vi "Log Errors.vi"(8 "error in (no error)":errorcluster, 11 "SV B-M (Host) in":refnum<class "SV B-M (Host).lvclass">) -> (0 "error out":errorcluster)   [LabVIEW 2015, in "SV B-M (Host).lvclass"]
doc: "Create an error log text file in the test directory that follows a template to record any error that occured during the benchmark sequence. If the error is known or expected, describe the error in detail."
uses:
  SV B-M (Host).lvclass
  SV B-M (Host).lvclass/SV B-M (Host).ctl
  Listbox - In Progress.vi
  Listbox - Complete.vi
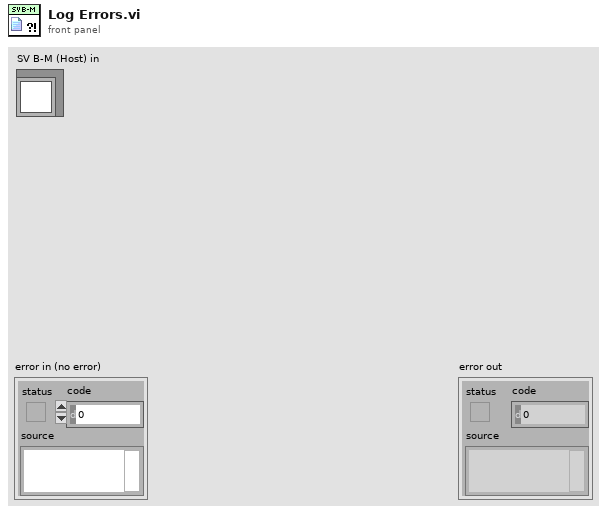
[diagram p1: front panel]
types:
  T1 = enum16{"open", "replace", "create", "open or create", "replace or create", "replace or create with confirmation"}
  T2 = typedef "Target Type.ctl" = enum16{"cRIO-9012", "cRIO-9014", "cRIO-9022", "cRIO-9023", "cRIO-9024", "cRIO-9025", "cRIO-9068", "cRIO-9073", "cRIO-9074", "cRIO-9075", "cRIO-9076", "cRIO-9081", "cRIO-9082", "myRIO-1900", "myRIO-1950", "PXI-8101", "PXI-8115", "PXI-8119", "PXI-8820", "PXIe-8100", "PXIe-8101", "PXIe-8133", "PXIe-8135", "PXIe-8820", "sbRIO-9605", "sbRIO-9606", "sbRIO-9623", "sbRIO-9626", "sbRIO-9633", "sbRIO-9636", "Unlisted (Linux-RT)", "Unlisted (PharLap)", "Unlisted (VxWorks)", "Windows Target"}
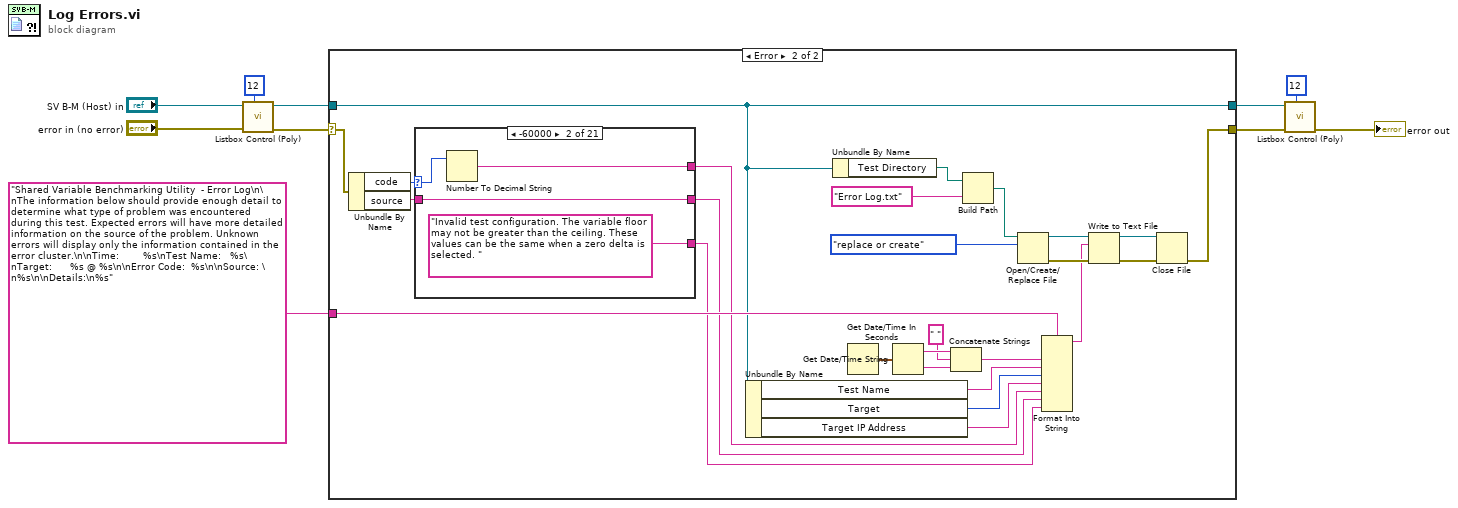
[diagram p0: block diagram]
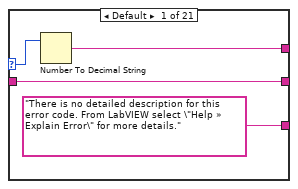
[diagram p3: hidden frame]
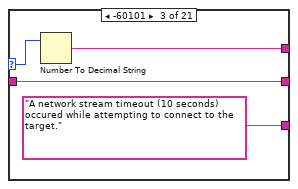
[diagram p4: hidden frame]
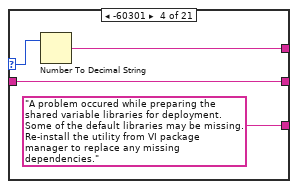
[diagram p5: hidden frame]
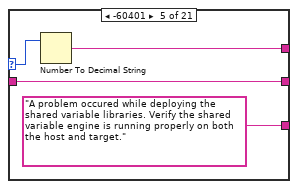
[diagram p6: hidden frame]
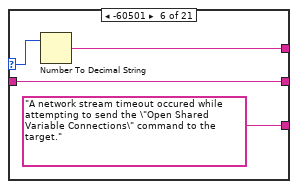
[diagram p7: hidden frame]
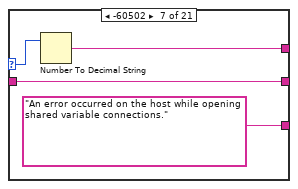
[diagram p8: hidden frame]
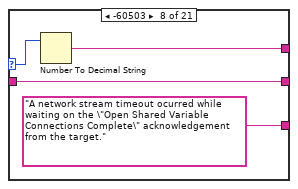
[diagram p9: hidden frame]
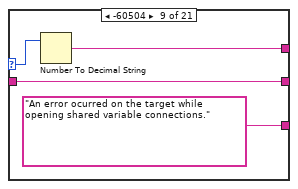
[diagram p10: hidden frame]
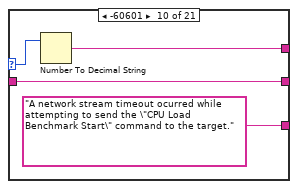
[diagram p11: hidden frame]
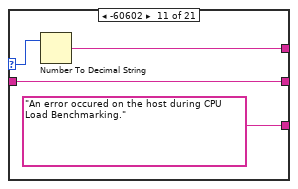
[diagram p12: hidden frame]
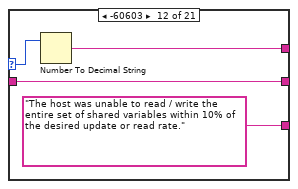
[diagram p13: hidden frame]
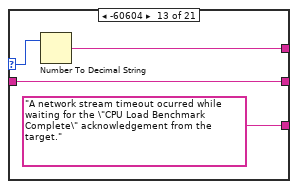
[diagram p14: hidden frame]
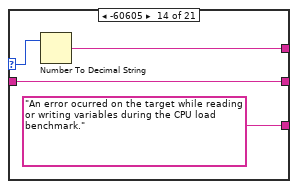
[diagram p15: hidden frame]
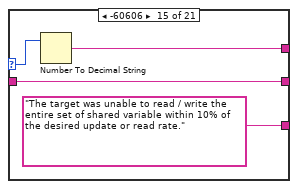
[diagram p16: hidden frame]
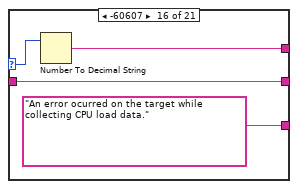
[diagram p17: hidden frame]
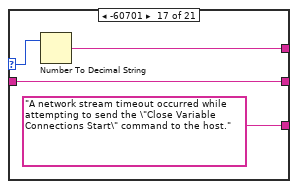
[diagram p18: hidden frame]
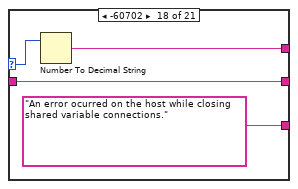
[diagram p19: hidden frame]
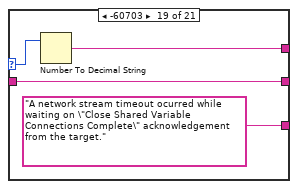
[diagram p20: hidden frame]
diagram:
  n1 = call-poly "Listbox Control (Poly).vi"("Row to Update"=12, "error in (no error)"="error in (no error)", "SV B-M In"="SV B-M (Host) in") -> ("error out"=w4:errorcluster, "SV B-M Out"=w5:refnum<class "SV B-M (Host).lvclass">)  [unwired: 7 in]
  n2 = case shown="Error" w4 {
    selector: w4 -> [w11 w18]
    tunnel: [w11 w20] -> w6
    tunnel: w5 -> [w12 w22]
    tunnel: [w12 w22] -> w3
    tunnel: "Shared Variable Benchmarking Utility  - Error Log\n\nThe information below should provide enough detail to determine what type of problem was encountered during this test. Expected errors will have more detailed information on the source of the problem. Unknown errors will display only the information contained in the error cluster.\n\nTime:        %s\nTest Name:   %s\nTarget:      %s @ %s\n\nError Code:  %s\n\nSource: \n%s\n\nDetails:\n%s" -> [_ w38]
    frame No Error {
    }
    frame Error {
      n3 = Unbundle By Name(w18) -> ("code"=w17:i32, "source"=w16:string)
      n4 = case shown="-60000" w17 {
        selector: w17 -> [w42 w46 w50 w54 w58 w62 w66 w70 w74 w78 w82 w86 w90 w94 w98 w102 w106 w110 w114 w118 w122]
        tunnel: w16 -> [w40 w44 w48 w52 w56 w60 w64 w68 w72 w76 w80 w84 w88 w92 w96 w100 w104 w108 w112 w116 w120]
        tunnel: [w41 w45 w49 w53 w57 w61 w65 w69 w73 w77 w81 w85 w89 w93 w97 w101 w105 w109 w113 w117 w121] -> w15
        tunnel: [w40 w44 w48 w52 w56 w60 w64 w68 w72 w76 w80 w84 w88 w92 w96 w100 w104 w108 w112 w116 w120] -> w14
        tunnel: ["There is no detailed description for this error code. From LabVIEW select \"Help » Explain Error\" for more details." "Invalid test configuration. The variable floor may not be greater than the ceiling. These values can be the same when a zero delta is selected. " "A network stream timeout (10 seconds) occured while attempting to connect to the target." "A problem occured while preparing the shared variable libraries for deployment. Some of the default libraries may be missing. Re-install the utility from VI package manager to replace any missing dependencies." "A problem occured while deploying the shared variable libraries. Verify the shared variable engine is running properly on both the host and target." "A network stream timeout occured while attempting to send the \"Open Shared Variable Connections\" command to the target." "An error occurred on the host while opening shared variable connections." "A network stream timeout ocurred while waiting on the \"Open Shared Variable Connections Complete\" acknowledgement from the target." "An error ocurred on the target while opening shared variable connections." "A network stream timeout ocurred while attempting to send the \"CPU Load Benchmark Start\" command to the target." "An error occured on the host during CPU Load Benchmarking." "The host was unable to read / write the entire set of shared variables within 10% of the desired update or read rate." "A network stream timeout ocurred while waiting for the \"CPU Load Benchmark Complete\" acknowledgement from the target." "An error ocurred on the target while reading or writing variables during the CPU load benchmark." "The target was unable to read / write the entire set of shared variable within 10% of the desired update or read rate." "An error ocurred on the target while collecting CPU load data." "A network stream timeout occurred while attempting to send the \"Close Variable Connections Start\" command to the host." "An error ocurred on the host while closing shared variable connections." "A network stream timeout ocurred while waiting on \"Close Shared Variable Connections Complete\" acknowledgement from the target." "An error occurred on the target while closing shared variable connections. Verify the shared variable engine on both the host and target is running properly." "An error ocurred while undeploying the shared variable libraries. Verify the shared variable engine is running properly on both the host and target."] -> w13
        frame Default {
          n5 = Number To Decimal String(number=w42) -> (decimal integer string=w41:string)  [unwired: 1 in]
        }
        frame -60000 {
          n6 = Number To Decimal String(number=w46) -> (decimal integer string=w45:string)  [unwired: 1 in]
        }
        frame -60101 {
          n7 = Number To Decimal String(number=w50) -> (decimal integer string=w49:string)  [unwired: 1 in]
        }
        frame -60301 {
          n8 = Number To Decimal String(number=w54) -> (decimal integer string=w53:string)  [unwired: 1 in]
        }
        frame -60401 {
          n9 = Number To Decimal String(number=w58) -> (decimal integer string=w57:string)  [unwired: 1 in]
        }
        frame -60501 {
          n10 = Number To Decimal String(number=w62) -> (decimal integer string=w61:string)  [unwired: 1 in]
        }
        frame -60502 {
          n11 = Number To Decimal String(number=w66) -> (decimal integer string=w65:string)  [unwired: 1 in]
        }
        frame -60503 {
          n12 = Number To Decimal String(number=w70) -> (decimal integer string=w69:string)  [unwired: 1 in]
        }
        frame -60504 {
          n13 = Number To Decimal String(number=w74) -> (decimal integer string=w73:string)  [unwired: 1 in]
        }
        frame -60601 {
          n14 = Number To Decimal String(number=w78) -> (decimal integer string=w77:string)  [unwired: 1 in]
        }
        frame -60602 {
          n15 = Number To Decimal String(number=w82) -> (decimal integer string=w81:string)  [unwired: 1 in]
        }
        frame -60603 {
          n16 = Number To Decimal String(number=w86) -> (decimal integer string=w85:string)  [unwired: 1 in]
        }
        frame -60604 {
          n17 = Number To Decimal String(number=w90) -> (decimal integer string=w89:string)  [unwired: 1 in]
        }
        frame -60605 {
          n18 = Number To Decimal String(number=w94) -> (decimal integer string=w93:string)  [unwired: 1 in]
        }
        frame -60606 {
          n19 = Number To Decimal String(number=w98) -> (decimal integer string=w97:string)  [unwired: 1 in]
        }
        frame -60607 {
          n20 = Number To Decimal String(number=w102) -> (decimal integer string=w101:string)  [unwired: 1 in]
        }
        frame -60701 {
          n21 = Number To Decimal String(number=w106) -> (decimal integer string=w105:string)  [unwired: 1 in]
        }
        frame -60702 {
          n22 = Number To Decimal String(number=w110) -> (decimal integer string=w109:string)  [unwired: 1 in]
        }
        frame -60703 {
          n23 = Number To Decimal String(number=w114) -> (decimal integer string=w113:string)  [unwired: 1 in]
        }
        frame -60704 {
          n24 = Number To Decimal String(number=w118) -> (decimal integer string=w117:string)  [unwired: 1 in]
        }
        frame -60801 {
          n25 = Number To Decimal String(number=w122) -> (decimal integer string=w121:string)  [unwired: 1 in]
        }
      }
      n26 = Unbundle By Name(w22) -> ("Test Name"=w32:string, "Target"=w31:T2, "Target IP Address"=w30:string)
      n27 = Unbundle By Name(w22) -> ("Test Directory"=w19:path)
      n28 = Get Date/Time In Seconds() -> (seconds since 1Jan1904=w37:timestamp)
      n29 = Get Date/Time String(seconds (now)=w37) -> (date string=w36:string, time string=w35:string)  [unwired: 2 in]
      n30 = Concatenate Strings(w36, " ", w35) -> (w33:string)
      n31 = Build Path(base path=w19, name or relative path="Error Log.txt") -> (appended path=w27:path)
      n32 = Open/Create/Replace File(file path (use dialog)=w27, operation (0:open)=T1."replace or create") -> (refnum out=w26:refnum<file>, error out=w25:errorcluster)  [unwired: 4 in, 1 out]
      n33 = Format Into String(format string=w38, w33, w32, w31, w30, w15, w14, w13) -> (resulting string=w21:string)  [unwired: 2 in, 1 out]
      n34 = Write to Text File(file (use dialog)=w26, text=w21, error in=w25) -> (refnum out=w24:refnum<file>, error out=w23:errorcluster)  [unwired: 1 in, 1 out]
      n35 = Close File(refnum=w24, error in=w23) -> (error out=w20:errorcluster)  [unwired: 1 out]
    }
  }
  n36 = call-poly "Listbox Control (Poly).vi"("Row to Update"=12, "error in (no error)"=w6, "SV B-M In"=w3) -> ("error out"=→"error out":errorcluster)  [unwired: 7 in, 1 out]
